vi "Reset.vi"(8 "error in (no error)":errorcluster, 11 "ATS9462 Class in":refnum<class "ATS9462 Class.lvclass">) -> (0 "error out":errorcluster, 3 "ATS9462 Class out":refnum<class "ATS9462 Class.lvclass">)   [LabVIEW 2014, in "ATS9462 Class.lvclass"]
uses:
  ATS9462 Class.lvclass
  ATS-VI/ATS_ctl/ATS_Async_Ctrl.ctl
  DAQ Class.lvclass
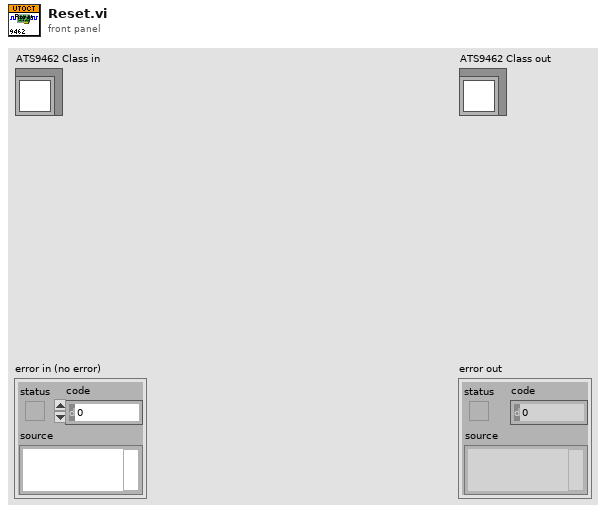
[diagram p1: front panel]
types:
  T1 = typedef "ATS_Async_Ctrl.ctl" = enum16{"SetupDMA", "StartCapture", "Get", "Get_Stream", "Abort", "Stop"}
  T2 = typedef "DAQ Class.lvclass/DAQ Parameters.ctl" = cluster{"Points Per A-Scan":u32, "A-Scans Per B-Scan":u32, "Number of B-Scans":u32, "A-Scans Per Transfer":u32, "Trigger Voltage":sgl, "Trigger Source":T3, "Trigger Slope":T4, "Channel":T5, "Clock":T6, "Bits per Sample":dbl, "Range":dbl}
  T3 = typedef "DAQ Class.lvclass/Trigger Source.ctl" = enum16{"External", "Channel A", "Channel B"}
  T4 = typedef "DAQ Class.lvclass/Trigger Slope.ctl" = enum16{"Rising", "Falling"}
  T5 = typedef "OCT DAQ Channel Data Type.ctl" = enum16{"Channel 1", "Channel 2", "Channel 1 and 2"}
  T6 = typedef "DAQ Class.lvclass/Clock Control.ctl" = enum16{"Internal Clock", "External Clock"}
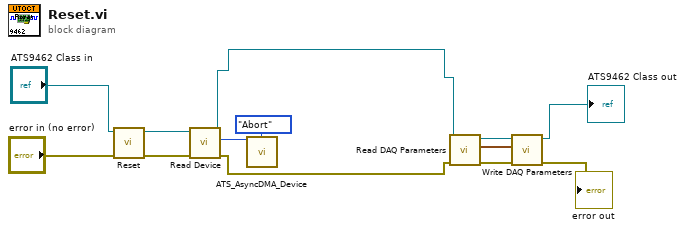
[diagram p0: block diagram]
diagram:
  n1 = call-parent "Reset.vi"("error in (no error)"="error in (no error)", "DAQ Class in"="ATS9462 Class in") -> ("error out"=w9:errorcluster, "DAQ Class out"=w10:refnum<class "ATS9462 Class.lvclass">)  [unwired: 8 in]
  n2 = call-dynamic "Read Device.vi"("error in (no error)"=w9, "ATS9462 Class in"=w10) -> ("error out"=w4:errorcluster, "Device"=w1:i32, "ATS9462 Class out"=w5:refnum<class "ATS9462 Class.lvclass">)  [unwired: 7 in]
  n3 = call "ATS_AsyncDMA_Device.vi"("DeviceIn"=w1, "ATS_Async_Ctrl"=ATS_Async_Ctrl."Abort") -> ()  [unwired: 9 in, 5 out]
  n4 = call-dynamic "Read DAQ Parameters.vi"("error in (no error)"=w4, "ATS9462 Class in"=w5) -> ("error out"=w6:errorcluster, "DAQ Parameters"=w7:T2, "ATS9462 Class out"=w8:refnum<class "ATS9462 Class.lvclass">)  [unwired: 7 in]
  n5 = call-dynamic "Write DAQ Parameters.vi"("error in (no error)"=w6, "DAQ Parameters"=w7, "ATS9462 Class in"=w8) -> ("error out"=→"error out":errorcluster, "ATS9462 Class out"=→"ATS9462 Class out":refnum<class "ATS9462 Class.lvclass">)  [unwired: 7 in]
